vi "Create Plugins.vi"(8 "error in (no error)":errorcluster, 9 "async plugins tag":string, 10 "inline plugins tag":string, 11 "Application Data In":T1) -> (0 "error out":errorcluster, 2 "avg bandwidth":dbl, 3 "Application Data out":T1)   [LabVIEW 2017, in "DSF Core.lvlib"]
uses:
  DSF Core.lvlib
  Main VI/Application Data.ctl
  <vilib>/NI/Memory Manager/Classes/Pointer/Pointer.lvclass
  Classes/Framework/Framework.lvclass
  Buffer Reader/Buffer Data.ctl
  Classes/Buffer/Buffer.lvclass
  C:/Program Files (x86)/National Instruments/LabVIEW 2017/vi.lib/NI/Memory Manager/Classes/Pointer/Pointer.lvclass
  Classes/Transfer Group Status/Status.lvclass
  Typedefs/DSF Engine Framework Configuration.ctl
  Typedefs/DSF Engine Plugin Configuration.ctl
  Typedefs/DSF Timing Info.ctl
  Typedefs/DSF Engine Plugin Thread Configuration.ctl
  Typedefs/DSF Settings Info.ctl
  Typedefs/DSF Engine Transfer Group Configuration.ctl
  Typedefs/DSF Direction.ctl
  Typedefs/DSF Engine Transfer Configuration.ctl
  Typedefs/DSF Byte Order.ctl
  Typedefs/DSF Engine Channel Configuration.ctl
  Typedefs/DSF Data Type.ctl
  Typedefs/DSF Timeout Behavior.ctl
  Classes/Framework/Framework.lvclass/Framework.ctl
  Classes/Framework Status/Framework Status.lvclass/Framework Status.ctl
  Classes/Plugin/Plugin.lvclass/Plugin.ctl
  Classes/Buffers/Buffers.lvclass/Buffers.ctl
  Classes/Timing/Timing.lvclass/Timing.ctl
  Classes/Transfer Group/Transfer Group.lvclass/Transfer Group.ctl
  <vilib>/NI/Memory Manager/Classes/Pointer/Pointer.lvclass/Pointer.ctl
  Classes/Transfer/Transfer.lvclass/Transfer.ctl
  Classes/Plugin/Get Name.vi
  Create New Tree Item.vi
  Add Transfer Group with Children.vi
  Classes/Plugin/Get Inline Tx Transfer Groups.vi
  Classes/Plugin/Get Async Rx Transfer Groups.vi
  Classes/Plugin/Get Async Tx Transfer Groups.vi
  Classes/Plugin/Get Inline Rx Transfer Groups.vi
  Classes/Plugin/Get Timing.vi
  Classes/Timing/Get Decimation.vi
  Classes/Plugin/Get Buffers.vi
  Classes/Buffers/Get String Buffer.vi
  Classes/Transfer Group/Get Name.vi
  Add Transfer.vi
  Classes/Transfer Group/Get Transfers.vi
  Classes/Transfer Group/Get Inline.vi
  Classes/Transfer Group/Get Timing.vi
  Classes/Transfer Group/Get Buffers.vi
  Buffer Reader/Average Cycle Bandwidth.vi
  Classes/Transfer/Get Name.vi
  Classes/Transfer/Get Buffers.vi
  Add Buffers.vi
  Classes/Buffer/Get Buffer Size.vi
  Classes/Buffers/Get Async Buffer.vi
  Classes/Buffers/Get Inline Buffer.vi
  <vilib>/NI/Memory Manager/Classes/Pointer/Get Size.vi
  Add Item to Tree.vi
  Classes/Framework Status/Framework Status.lvclass
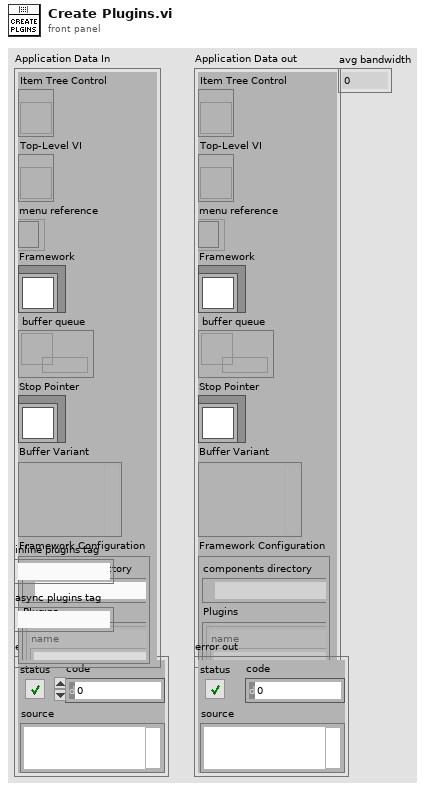
[diagram p1: front panel]
types:
  T1 = typedef "DSF Core.lvlib/Application Data.ctl" = cluster{"Item Tree Control":refnum<vi>, "Top-Level VI":refnum<vi>, "menu reference":refnum<k9>, "Framework":refnum<class "Framework.lvclass">, "buffer queue":refnum<queue>, "Stop Pointer":refnum<class "Pointer.lvclass">, "Buffer Variant":variant, "Framework Configuration":T2}
  T2 = typedef "DSF Core.lvlib/DSF Engine Framework Configuration.ctl" = cluster{"components directory":path, "Plugins":T3[]}
  T3 = typedef "DSF Core.lvlib/DSF Engine Plugin Configuration.ctl" = cluster{"name":string, "components":string[], "cycle timing":T4, "threads":T5[], "Transfer Groups":T7[], "settings":T6}
  T4 = typedef "DSF Core.lvlib/DSF Timing Info.ctl" = cluster{"priority":u64, "decimation":u64, "offset":u64}
  T5 = typedef "DSF Core.lvlib/DSF Engine Plugin Thread Configuration.ctl" = cluster{"buffer converter settings":T6, "transceiver settings":T6, "processor":i32, "priority offset":i16}
  T6 = typedef "DSF Core.lvlib/DSF Settings Info.ctl" = cluster{"key":string, "value":string}[]
  T7 = typedef "DSF Core.lvlib/DSF Engine Transfer Group Configuration.ctl" = cluster{"name":string, "direction":T8, "cycle timing":T4, "thread index":i32, "settings":T6, "Transfers":T9[], "timeout behavior":T13}
  T8 = typedef "DSF Core.lvlib/DSF Direction.ctl" = enum8{"Tx", "Rx"}
  T9 = typedef "DSF Core.lvlib/DSF Engine Transfer Configuration.ctl" = cluster{"name":string, "byte order":T10, "settings":T6, "channels":T11[]}
  T10 = typedef "DSF Core.lvlib/DSF Byte Order.ctl" = enum8{"big-endian", "little-endian"}
  T11 = typedef "DSF Core.lvlib/DSF Engine Channel Configuration.ctl" = cluster{"string offset":u64, "string data type":T12, "engine data type":T12, "name":string, "settings":T6}
  T12 = typedef "DSF Core.lvlib/DSF Data Type.ctl" = enum8{"Bool", "SGL", "DBL", "I8", "I16", "I32", "I64", "U8", "U16", "U32", "U64"}
  T13 = typedef "DSF Core.lvlib/DSF Timeout Behavior.ctl" = enum8{"Increment Late Count", "Throw Error"}
  T14 = typedef "DSF Core.lvlib/Buffer Data.ctl" = cluster{"Buffer":refnum<class "Buffer.lvclass">, "Status":refnum<class "Status.lvclass">, "decimation":u64, "avg bandwidth":dbl}
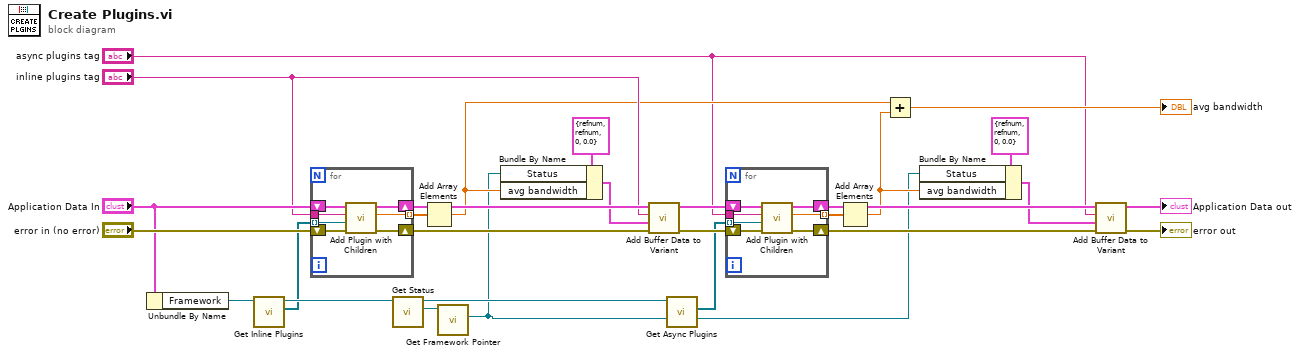
[diagram p0: block diagram]
diagram:
  n1 = Unbundle By Name("Application Data In") -> ("Framework"=w5:refnum<class "Framework.lvclass">)
  n2 = call "Get Inline Plugins.vi"("Framework in"=w5) -> ("Inline Plugins"=w3:refnum<class "Plugin.lvclass">[], "Framework out"=w4:refnum<class "Framework.lvclass">)  [unwired: 9 in]
  n3 = for {
    shift-right: [w32] -> w22
    shift-left: "error in (no error)" -> [w34]
    tunnel: w3 -> [w30] mode=indexing
    tunnel: "inline plugins tag" -> [w31]
    shift-right: [w33] -> w23
    shift-left: "Application Data In" -> [w35]
    tunnel: [w29] -> w26 mode=indexing
    n4 = call "Add Plugin with Children.vi"("error in (no error)"=w34, "Plugin"=w30, "parent tag"=w31, "Application Data In"=w35) -> ("error out"=w32:errorcluster, "average bandwidth"=w29:dbl, "Application Data Out"=w33:T1)  [unwired: 5 in]
  }
  n5 = call "Get Status.vi"("Framework in"=w4) -> ("Status"=w7:refnum<class "Framework Status.lvclass">, "Framework out"=w2:refnum<class "Framework.lvclass">)  [unwired: 9 in]
  n6 = Add Array Elements(numeric array=w26) -> (sum=w12:dbl)
  n7 = call "Get Framework Pointer.vi"("Framework Status in"=w7) -> ("framework pointer"=w1:refnum<class "Status.lvclass">)  [unwired: 9 in, 1 out]
  n8 = Bundle By Name(cluster=T14 {"Buffer"=refnum, "Status"=refnum, "decimation"=0, "avg bandwidth"=0.0} ("Buffer data"), "Status"=w1, "avg bandwidth"=w12) -> (w13:T14)
  n9 = call "Add Buffer Data to Variant.vi"("error in (no error)"=w22, "Buffer data"=w13, "tag"="inline plugins tag", "Application Data In in"=w23) -> ("error out"=w20:errorcluster, "Application Data In out"=w21:T1)  [unwired: 6 in]
  n10 = call "Get Async Plugins.vi"("Framework in"=w2) -> ("Async Plugins"=w11:refnum<class "Plugin.lvclass">[])  [unwired: 9 in, 1 out]
  n11 = for {
    shift-right: [w39] -> w17
    shift-left: w20 -> [w41]
    shift-right: [w40] -> w19
    shift-left: w21 -> [w42]
    tunnel: "async plugins tag" -> [w38]
    tunnel: w11 -> [w37] mode=indexing
    tunnel: [w36] -> w25 mode=indexing
    n12 = call "Add Plugin with Children.vi"("error in (no error)"=w41, "Plugin"=w37, "parent tag"=w38, "Application Data In"=w42) -> ("error out"=w39:errorcluster, "average bandwidth"=w36:dbl, "Application Data Out"=w40:T1)  [unwired: 5 in]
  }
  n13 = Add Array Elements(numeric array=w25) -> (sum=w9:dbl)
  n14 = Add(x=w12, y=w9) -> (x+y=→"avg bandwidth":dbl)
  n15 = Bundle By Name(cluster=T14 {"Buffer"=refnum, "Status"=refnum, "decimation"=0, "avg bandwidth"=0.0} ("Buffer data"), "Status"=w1, "avg bandwidth"=w9) -> (w8:T14)
  n16 = call "Add Buffer Data to Variant.vi"("error in (no error)"=w17, "Buffer data"=w8, "tag"="async plugins tag", "Application Data In in"=w19) -> ("error out"=→"error out":errorcluster, "Application Data In out"=→"Application Data out":T1)  [unwired: 6 in]
